vi "Translation_Equals.vi"(9 "other Translation":T1, 11 "In Translation":T1) -> (3 "Equals":bool)   [LabVIEW 2019, in "Trajectory_Library.lvlib"]
doc: "Checks equality between this Translation2d and another object.\n\nParameters:\n - IN TRANSLATION - This TRANSLATION data structure\n - OTHER TRANSLATION - The other TRANSLATION data structure\n\nReturns:\n - EQUALS - Value is set to TRUE if the two TRANSLATIONS are equal."
uses:
  Trajectory_Library.lvlib
  TRANSLATION2D.ctl
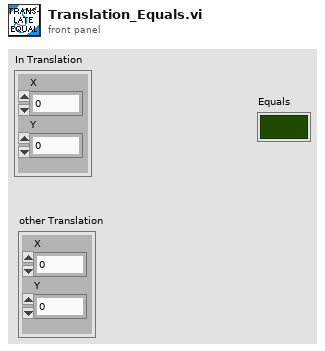
[diagram p1: front panel]
types:
  T1 = typedef "Trajectory_Library.lvlib/TRANSLATION2D.ctl" = cluster{"X":dbl, "Y":dbl}
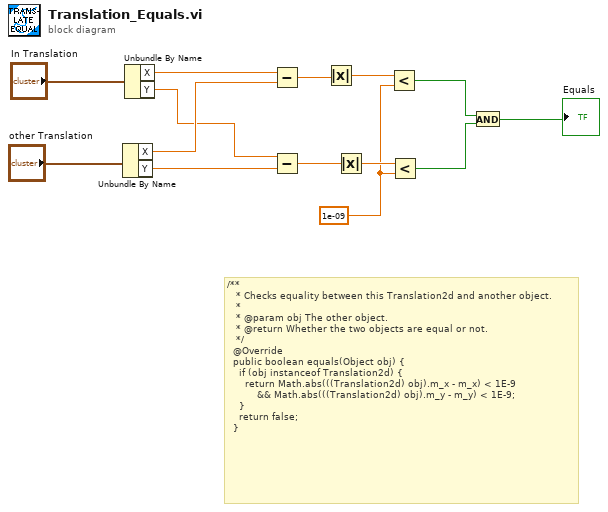
[diagram p0: block diagram]
diagram:
  w4 = 1e-09 ("y")
  # "/**\n   * Checks equality between this Translation2d and another object.\n   *\n   * @param obj The other object.\n   * @return Whether the two objects are equal or not.\n   */\n  @Override\n  public boolean equals(Object obj) {\n    if (obj instanceof Translation2d) {\n      return Math.abs(((Translation2d) obj).m_x - m_x) < 1E-9\n          && Math.abs(((Translation2d) obj).m_y - m_y) < 1E-9;\n    }\n    return false;\n  }"
  n1 = Unbundle By Name("other Translation") -> ("X"=w11:dbl, "Y"=w10:dbl)
  n2 = Unbundle By Name("In Translation") -> ("X"=w12:dbl, "Y"=w9:dbl)
  n3 = Subtract(x=w12, y=w11) -> (x-y=w7:dbl)
  n4 = Subtract(x=w9, y=w10) -> (x-y=w8:dbl)
  n5 = Absolute Value(x=w7) -> (abs(x)=w5:dbl)
  n6 = Absolute Value(x=w8) -> (abs(x)=w6:dbl)
  n7 = Less?(x=w5, y=w4) -> (x < y?=w3:bool)
  n8 = Less?(x=w6, y=w4) -> (x < y?=w2:bool)
  n9 = And(x=w3, y=w2) -> (x .and. y?=→"Equals":bool)
